vi "Open Server Connection.vi"(8 "error in (no error)":errorcluster, 9 "port":u16, 10 "address":string, 11 "RemoteControl.ZMQ in":refnum<class "RemoteControl.ZMQ.lvclass">) -> (0 "error out":errorcluster, 3 "RemoteControl.ZMQ out":refnum<class "RemoteControl.ZMQ.lvclass">)   [LabVIEW 2019, in "RemoteControl.ZMQ.lvlib" / "RemoteControl.ZMQ.lvclass"]
uses:
  RemoteControl.ZMQ.lvclass
  <vilib>/addons/zeromq/socket_type.ctl
  RemoteControl.ZMQ.lvclass/RemoteControl.ZMQ.ctl
  <userlib>/LevyLab/RemoteControl/RemoteControl/RemoteControl.lvclass
  <vilib>/addons/zeromq/zeromq.lvlib
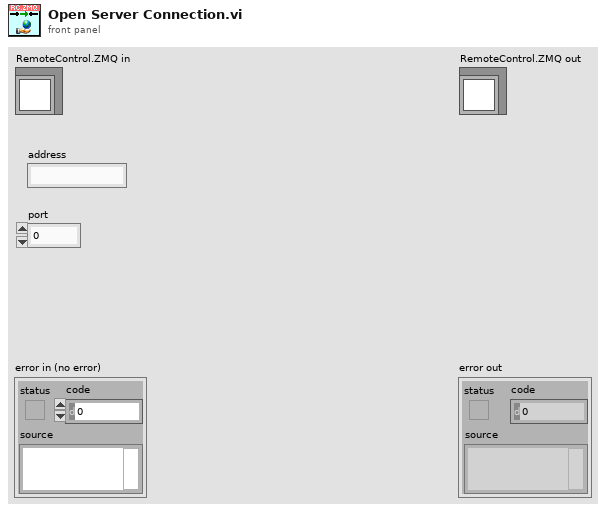
[diagram p1: front panel]
types:
  T1 = typedef "zeromq.lvlib/socket_type.ctl" = enum8{"ZMQ_PAIR", "ZMQ_PUB", "ZMQ_SUB", "ZMQ_REQ", "ZMQ_REP", "ZMQ_DEALER", "ZMQ_ROUTER", "ZMQ_PULL", "ZMQ_PUSH", "ZMQ_XPUB", "ZMQ_XSUB", "ZMQ_STREAM", "ZMQ_SERVER", "ZMQ_CLIENT", "ZMQ_RADIO", "ZMQ_DISH", "ZMQ_GATHER", "ZMQ_SCATTER", "ZMQ_DGRAM"}
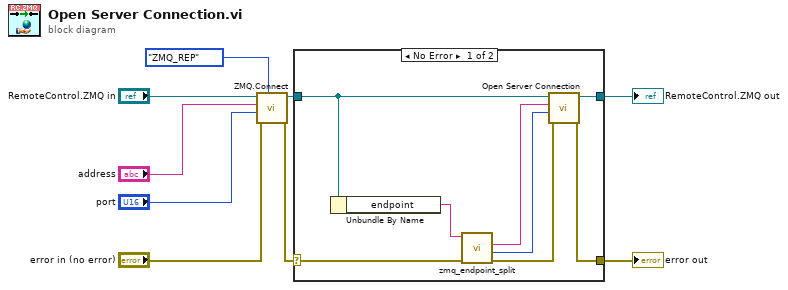
[diagram p0: block diagram]
diagram:
  n1 = call "ZMQ.Connect.vi"("socket type"=socket_type."ZMQ_REP", "error in (no error)"="error in (no error)", "port"="port", "address"="address", "RemoteControl.ZMQ in"="RemoteControl.ZMQ in") -> ("error out"=w6:errorcluster, "RemoteControl.ZMQ out"=w5:refnum<class "RemoteControl.ZMQ.lvclass">)  [unwired: 5 in]
  n2 = case shown="No Error" w6 {
    selector: w6 -> [w14 w18]
    tunnel: w5 -> [w12 w19]
    tunnel: [w11 w19] -> w4
    tunnel: [w10 w18] -> w3
    frame No Error {
      n3 = Unbundle By Name(w12) -> ("endpoint"=w15:string)
      n4 = call <vilib>:"zmq_endpoint_split.vi"("error in"=w14, "endpoint"=w15) -> ("error out"=w13:errorcluster, "port"=w16:u16, "address"=w17:string)  [unwired: 2 in, 1 out]
      n5 = call-parent "Open Server Connection.vi"("error in (no error)"=w13, "Port"=w16, "address"=w17, "RemoteControl in"=w12) -> ("error out"=w10:errorcluster, "RemoteControl out"=w11:refnum<class "RemoteControl.ZMQ.lvclass">)  [unwired: 6 in]
    }
    frame Error {
    }
  }
  "error out" <- w3
  "RemoteControl.ZMQ out" <- w4
